vi "get analog value .vi"(10 "pin":i32, 11 "daq":u32) -> (2 "function return":dbl, 3 "daq out":u32)   [LabVIEW 2020, in "cDaq.lvlib"]
doc: "DAQAPI double get_analog_value_(HDAQ daq, int pin);"
uses:
  cDaq.lvlib
  <userlib>/cDaq/cDaq.dll
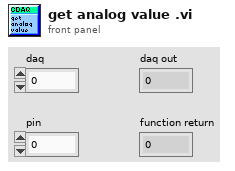
[diagram p1: front panel]
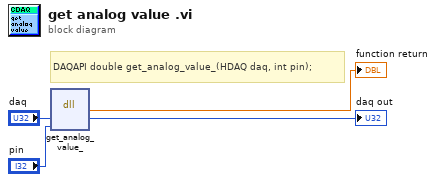
[diagram p0: block diagram]
diagram:
  # "DAQAPI double get_analog_value_(HDAQ daq, int pin);"
  n1 = dll-call lib="C:/Program Files (x86)/National Instruments/LabVIEW 2020/user.lib/cDaq/cDaq.*" fn="get_analog_value_"("daq"="daq", "pin"="pin") -> ("type de retour"=→"function return":dbl, "daq"=→"daq out":u32)  [unwired: 4 in, 2 out]
